vi "BigExtendedEuclidean.vi"(1 "b":cluster{"Boolean":bool, "Array":u64[]}, 2 "a":cluster{"Boolean":bool, "Array":u64[]}) -> (0 "c (ac mod(b) = 1)":cluster{"Boolean":bool, "Array":u64[]})   [LabVIEW 2023]
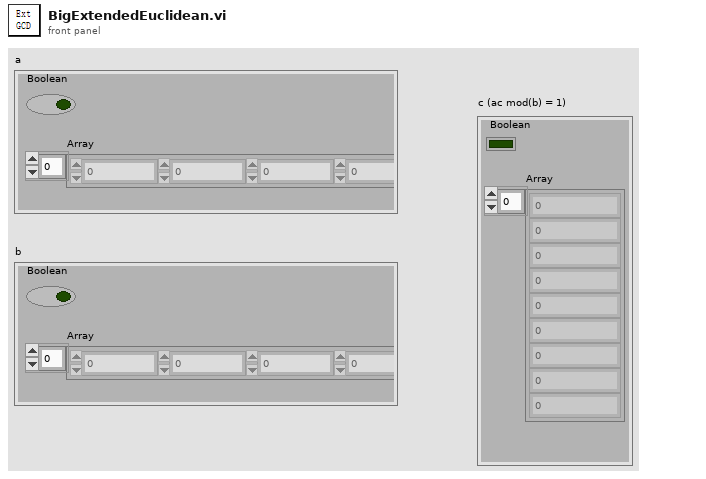
[diagram p1: front panel]
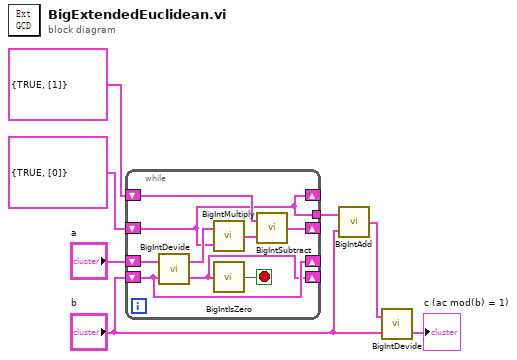
[diagram p0: block diagram]
diagram:
  n1 = while {
    shift-right: [w14] -> _
    shift-left: "b" -> [w15]
    shift-right: [w15] -> _
    shift-left: "a" -> [w16]
    shift-right: [w8] -> _
    shift-left: cluster{bool, u64[]} {TRUE, [1]} -> [w12]
    shift-right: [w9] -> _
    shift-left: cluster{bool, u64[]} {TRUE, [0]} -> [w8]
    tunnel: [w8] -> w4
    stop <- w13 stop-if-true
    n2 = call "BigIntDevide.vi"("b"=w15, "a"=w16) -> ("a % b"=w14:cluster{"Boolean":bool, "Array":u64[]}, "a / b"=w11:cluster{"Boolean":bool, "Array":u64[]})
    n3 = call "BigIntMultiply.vi"("b"=w8, "a"=w11) -> ("a * b"=w10:cluster{"Boolean":bool, "Array":u64[]})
    n4 = call "BigIntIsZero.vi"("a"=w14) -> ("a = 0"=w13:bool)
    n5 = call "BigIntSubtract.vi"("b"=w10, "a"=w12) -> ("a - b"=w9:cluster{"Boolean":bool, "Array":u64[]})
  }
  n6 = call "BigIntAdd.vi"("b"="b", "a"=w4) -> ("a + b"=w3:cluster{"Boolean":bool, "Array":u64[]})
  n7 = call "BigIntDevide.vi"("b"="b", "a"=w3) -> ("a % b"=→"c (ac mod(b) = 1)":cluster{"Boolean":bool, "Array":u64[]})  [unwired: 1 out]
